vi "Consumer Console Entry.vi"(0 "Consumer Data In":T2={"Queue_Consumer"=refnum, "Selected Consumer"=enum."Random", "Session Data"={"Tx-Data"=[], "Rx-Data"=[], "MIDI-Message log"=[{"Message Name"="", "Meta value"=0, "Datastring"="", "Datatype"=enum."No Data"}]}, "Timout-Time[ms]"=0, "To_GUI-Consumer"=refnum, "CPU(ms)"=0, "Console log"="", "MIDI Parse Data"={"MIDI-Bytes In"=[145, 60, 100], "MIDI Tag"=[], "MIDI Parsed Data"=[], "Iteration"=0, "Error?"=[], "Running States"=[], "Running Statusbyte"=0, "Running StatusString"="", "Third Byte Flag"=FALSE, "Current Byte"=0, "Sysex"="", "Expect Databyte"=FALSE}, "Session Inspection Data"={"Diff"=[], "Tx Byte"=[], "Rx Byte"=[], "Send Log"=[], "Parsed Data"={"Tx MIDI Tag"=[], "Tx MIDI Parsed Data"=[], "Tx Error"=[], "Tx Running States"=[], "Rx MIDI Tag"=[], "Rx MIDI Parsed Data"=[], "Rx Error"=[], "Rx Running States"=[], "Diff"=[]}}} {"MIDI Parse Data"."Current Byte" format="%.0x"; "MIDI Parse Data"."Running Statusbyte" format="%.0x"; "MIDI Parse Data"."MIDI-Bytes In" format="%.0x"}, 11 "Console Entry":string, 13 "Error In":errorcluster) -> (4 "Consumer Data Out":T2={"Queue_Consumer"=refnum, "Selected Consumer"=enum."Random", "Session Data"={"Tx-Data"=[], "Rx-Data"=[], "MIDI-Message log"=[{"Message Name"="", "Meta value"=0, "Datastring"="", "Datatype"=enum."No Data"}]}, "Timout-Time[ms]"=0, "To_GUI-Consumer"=refnum, "CPU(ms)"=0, "Console log"="", "MIDI Parse Data"={"MIDI-Bytes In"=[145, 60, 100], "MIDI Tag"=[], "MIDI Parsed Data"=[], "Iteration"=0, "Error?"=[], "Running States"=[], "Running Statusbyte"=0, "Running StatusString"="", "Third Byte Flag"=FALSE, "Current Byte"=0, "Sysex"="", "Expect Databyte"=FALSE}, "Session Inspection Data"={"Diff"=[], "Tx Byte"=[], "Rx Byte"=[], "Send Log"=[], "Parsed Data"={"Tx MIDI Tag"=[], "Tx MIDI Parsed Data"=[], "Tx Error"=[], "Tx Running States"=[], "Rx MIDI Tag"=[], "Rx MIDI Parsed Data"=[], "Rx Error"=[], "Rx Running States"=[], "Diff"=[]}}} {"MIDI Parse Data"."Current Byte" format="%.0x"; "MIDI Parse Data"."Running Statusbyte" format="%.0x"; "MIDI Parse Data"."MIDI-Bytes In" format="%.0x"})   [LabVIEW 2019]
doc: "Adds a new entry to a console log, if an error has occured it will also be logged."
uses:
  Controls/Consumer_Data.ctl
  Common/Controls/Application_Message.ctl
  Common/Controls/Application_State.ctl
  Controls/Consumer_States.ctl
  Controls/Transfer_Data.ctl
  MIDI/Controls/MIDI-Message_Array.ctl
  MIDI/Controls/MIDI-Message_Cluster.ctl
  MIDI/Controls/Meta_Commands.ctl
  Controls/Parser-data.ctl
  Controls/Consumer_Result.ctl
  Controls/Parsed_Data.ctl
panel:
  in  "Tab Control":T1(tab)
  out "Console log in":string
  out "Timestamp":string
  out "Console log out":string
  out "VI-filename":string
  out "VI Path":path
  out "Code Size":u32
  out "Revision Number":u32
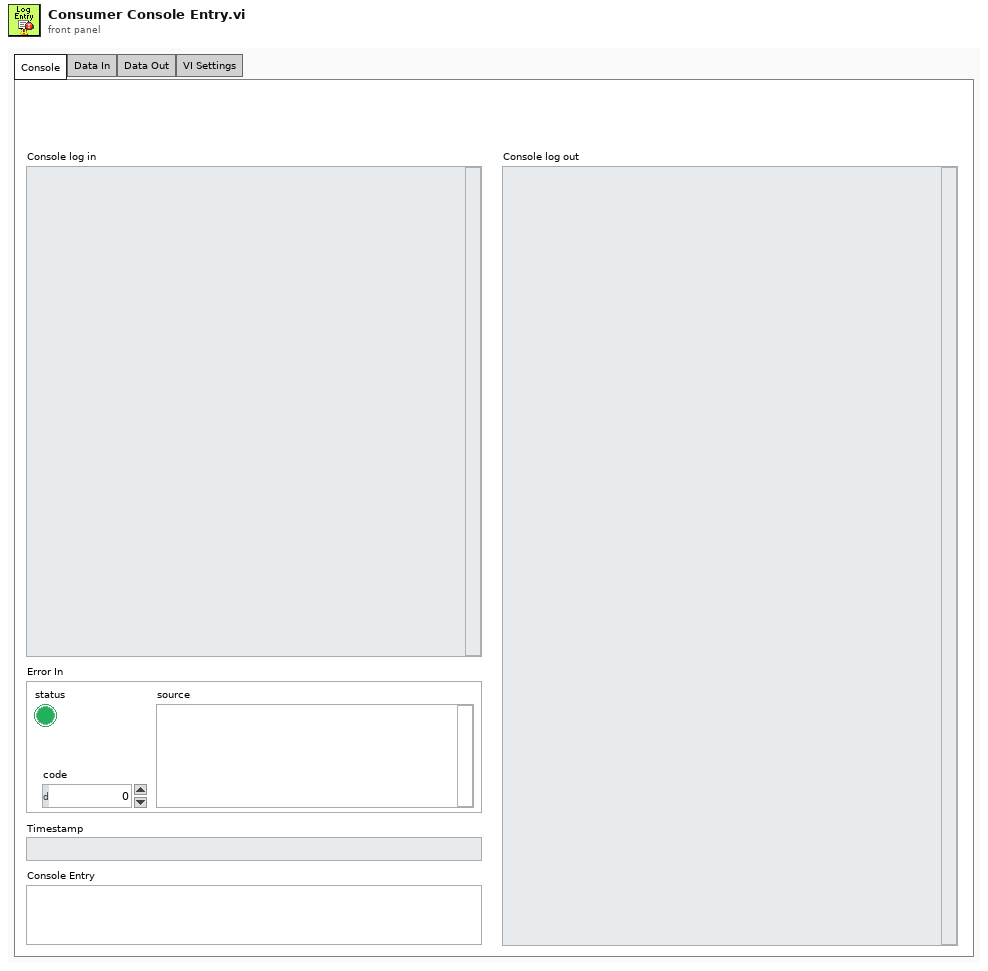
[diagram p1: front panel]
types:
  T1 = enum32{"Console", "Data In", "Data Out", "VI Settings"}
  T2 = typedef "Consumer_Data.ctl" = cluster{"Queue_Consumer":refnum<queue>, "Selected Consumer":T3, "Session Data":T4, "Timout-Time[ms]":i32, "To_GUI-Consumer":refnum<user-event>, "CPU(ms)":u32, "Console log":string, "MIDI Parse Data":T8, "Session Inspection Data":T9}
  T3 = typedef "Consumer_States.ctl" = enum16{"Random", "ECG", "Strech-Patch"}
  T4 = typedef "Transfer_Data.ctl" = cluster{"Tx-Data":i8[], "Rx-Data":i8[], "MIDI-Message log":T5}
  T5 = typedef "MIDI-Message_Array.ctl" = T6[]
  T6 = typedef "MIDI-Message_Cluster.ctl" = cluster{"Message Name":string, "Meta value":i32, "Datastring":string, "Datatype":T7}
  T7 = typedef "Meta_Commands.ctl" = enum16{"No Data", "Pause", "Loop", "Wait for Rx", "Delay", "Break", "MIDI"}
  T8 = typedef "Parser-data.ctl" = cluster{"MIDI-Bytes In":u8[], "MIDI Tag":string[], "MIDI Parsed Data":string[], "Iteration":i32, "Error?":bool[], "Running States":string[], "Running Statusbyte":u8, "Running StatusString":string, "Third Byte Flag":bool, "Current Byte":u8, "Sysex":string, "Expect Databyte":bool}
  T9 = typedef "Consumer_Result.ctl" = cluster{"Diff":bool[], "Tx Byte":string[], "Rx Byte":string[], "Send Log":string[], "Parsed Data":T10}
  T10 = typedef "Parsed_Data.ctl" = cluster{"Tx MIDI Tag":string[], "Tx MIDI Parsed Data":string[], "Tx Error":bool[], "Tx Running States":string[], "Rx MIDI Tag":string[], "Rx MIDI Parsed Data":string[], "Rx Error":bool[], "Rx Running States":string[], "Diff":bool[]}
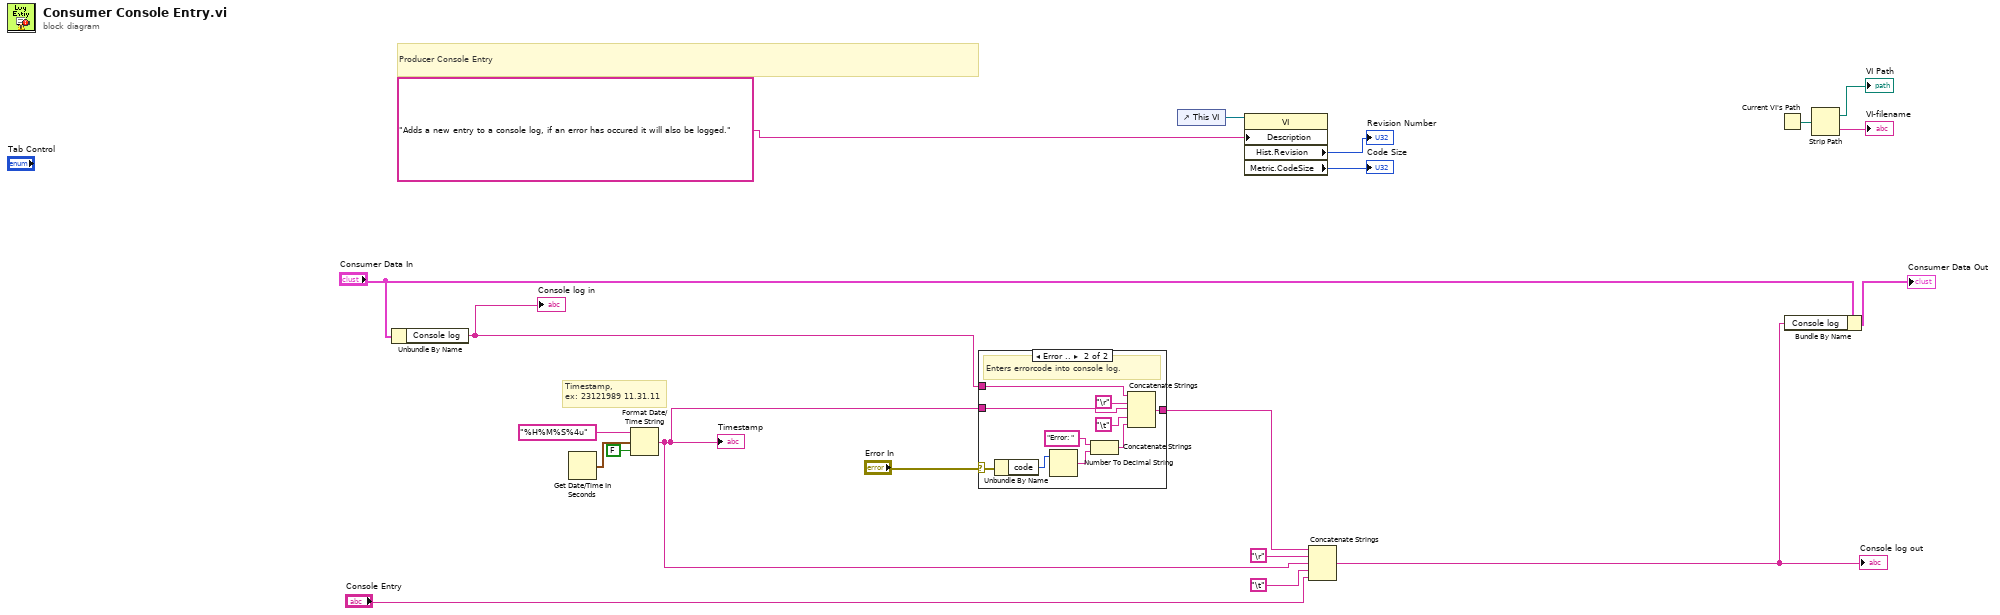
[diagram p0: block diagram]
diagram:
  # "Timestamp, \nex: 23121989 11.31.11"
  # "Producer Console Entry"
  n1 = Unbundle By Name("Consumer Data In") -> ("Console log"=w9:string)
  "Console log in" <- w9
  n2 = Get Date/Time In Seconds() -> (seconds since 1Jan1904=w13:timestamp)
  n3 = Format Date/Time String(time format string (%c)="%H%M%S%4u", seconds (now)=w13, UTC format=FALSE) -> (date/time string=w8:string)
  "Timestamp" <- w8
  n4 = case shown="Error .." "Error In" {
    selector: "Error In" -> [_ w22]
    tunnel: w9 -> [w21 w27]
    tunnel: w8 -> [_ w25]
    tunnel: [w21 w23] -> w7
    frame No Error {
    }
    frame Error {
      # "Enters errorcode into console log."
      n5 = Unbundle By Name(w22) -> ("code"=w31:i32)
      n6 = Number To Decimal String(number=w31) -> (decimal integer string=w30:string)  [unwired: 1 in]
      n7 = Concatenate Strings("Error: " ("string"), w30) -> (w29:string)
      n8 = Concatenate Strings(w27, "\r", w25, "\t", w29) -> (w23:string)
    }
  }
  n9 = control-ref of="This VI"() -> (w4:refnum<vi>)
  n10 = property class="VI"(reference=w4, "Description"="Adds a new entry to a console log, if an error has occured it will also be logged.") -> ("Hist.Revision"=→"Revision Number":u32, "Metric.CodeSize"=→"Code Size":u32)  [unwired: 1 in, 2 out]
  n11 = Concatenate Strings(w7, "\r", w8, "\t", "Console Entry") -> (w16:string)
  "Console log out" <- w16
  n12 = Current VI's Path() -> (path=w20:path)
  n13 = Bundle By Name(cluster="Consumer Data In", "Console log"=w16) -> (→"Consumer Data Out":T2)
  n14 = Strip Path(path=w20) -> (stripped path=→"VI Path":path, name=→"VI-filename":string)
